vi "WMI DOTNET.vi"() -> ()   [LabVIEW 2017]
uses:
  System.Management
panel:
  out "TotalPhysicalMemory":i32[](array[numeric])
  out "Array":string[](array[string])
  out "Current":refnum<k24>
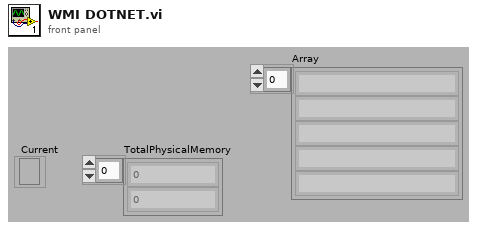
[diagram p1: front panel]
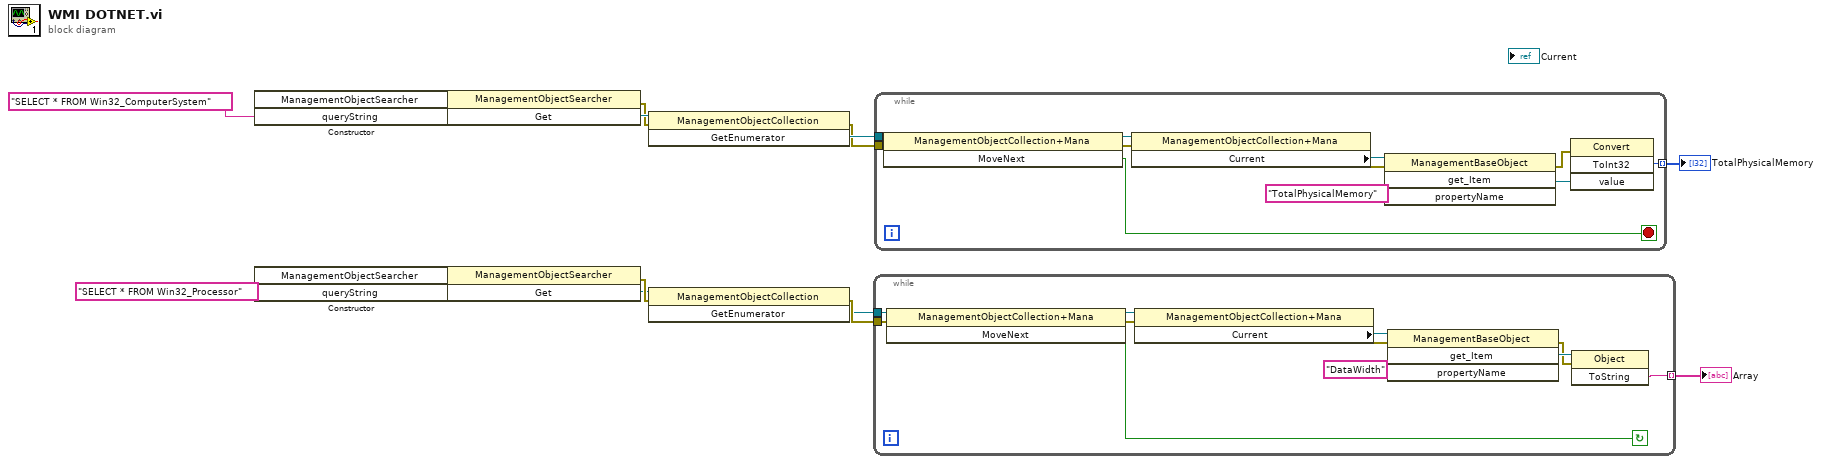
[diagram p0: block diagram]
diagram:
  n1 = constructor class="ManagementObjectSearcher"("queryString"="SELECT * FROM Win32_ComputerSystem") -> (reference out=w14:refnum<k24>, error out=w13:errorcluster)  [unwired: 3 in, 2 out]
  n2 = constructor class="ManagementObjectSearcher"("queryString"="SELECT * FROM Win32_Processor") -> (reference out=w5:refnum<k24>, error out=w6:errorcluster)  [unwired: 3 in, 2 out]
  n3 = invoke class="ManagementObjectSearcher" method="Get"(reference=w14, error in=w13) -> (error out=w12:errorcluster, "Get"=w16:refnum<k24>)  [unwired: 1 in, 1 out]
  n4 = invoke class="ManagementObjectSearcher" method="Get"(reference=w5, error in=w6) -> (error out=w7:errorcluster, "Get"=w3:refnum<k24>)  [unwired: 1 in, 1 out]
  n5 = invoke class="ManagementObjectCollection" method="GetEnumerator"(reference=w16, error in=w12) -> (error out=w10:errorcluster, "GetEnumerator"=w11:refnum<k24>)  [unwired: 1 in, 1 out]
  n6 = invoke class="ManagementObjectCollection" method="GetEnumerator"(reference=w3, error in=w7) -> (error out=w9:errorcluster, "GetEnumerator"=w8:refnum<k24>)  [unwired: 1 in, 1 out]
  n7 = while {
    tunnel: w9 -> [w26]
    tunnel: w8 -> [w24]
    tunnel: [w17] -> w2 mode=indexing
    stop <- w20 continue-if-true
    n8 = invoke class="ManagementObjectCollection+Mana" method="MoveNext"(reference=w24, error in=w26) -> (reference out=w25:refnum<k24>, error out=w27:errorcluster, "MoveNext"=w20:bool)  [unwired: 1 in]
    n9 = property class="ManagementObjectCollection+Mana"(reference=w25, error in=w27) -> (error out=w23:errorcluster, "Current"=w21:refnum<k24>)  [unwired: 1 out]
    n10 = invoke class="ManagementBaseObject" method="get_Item"(reference=w21, error in=w23, "propertyName"="DataWidth") -> (error out=w18:errorcluster, "get_Item"=w19:refnum<k24>)  [unwired: 1 in, 2 out]
    n11 = invoke class="Object" method="ToString"(reference=w19, error in=w18) -> ("ToString"=w17:string)  [unwired: 1 in, 2 out]
  }
  "Array" <- w2
  n12 = while {
    tunnel: [w35] -> w1 mode=indexing
    tunnel: w11 -> [w33]
    tunnel: w10 -> [w31]
    stop <- w28 stop-if-true
    n13 = invoke class="ManagementObjectCollection+Mana" method="MoveNext"(reference=w33, error in=w31) -> (reference out=w32:refnum<k24>, error out=w30:errorcluster, "MoveNext"=w28:bool)  [unwired: 1 in]
    n14 = property class="ManagementObjectCollection+Mana"(reference=w32, error in=w30) -> (error out=w34:errorcluster, "Current"=w38:refnum<k24>)  [unwired: 1 out]
    n15 = invoke class="ManagementBaseObject" method="get_Item"(reference=w38, error in=w34, "propertyName"="TotalPhysicalMemory") -> (error out=w29:errorcluster, "get_Item"=w36:refnum<k24>)  [unwired: 1 in, 2 out]
    n16 = invoke class="Convert" method="ToInt32"(error in=w29, "value"=w36) -> ("ToInt32"=w35:i32)  [unwired: 2 in, 3 out]
  }
  "TotalPhysicalMemory" <- w1
